vi "System_Data_Save.vi"(8 "error in":errorcluster, 11 "System Data":T1={"System"={"Active"=FALSE, "Exit"=FALSE, "Command wait"="", "Status_Time"=0, "Time_GPS"=0}, "Stepper Motor"={"Connection Reference"="", "Valid Connection"=FALSE, "Speed"=15}, "Camera Data"={"Image path"=path "", "Filenames"=[], "Filenames queue"=[]}, "Core"={"Close Panel on Exit?"=FALSE, "Current VI Reference"=refnum}} {"Stepper Motor"."Speed" scale=0.0..30.0}) -> (0 "error out":errorcluster, 3 "path":path)   [LabVIEW 2019]
uses:
  System Data.ctl
  Stepper Data.ctl
  Camera Data.ctl
  <vilib>/Utility/xml.llb/Write to XML File(string).vi
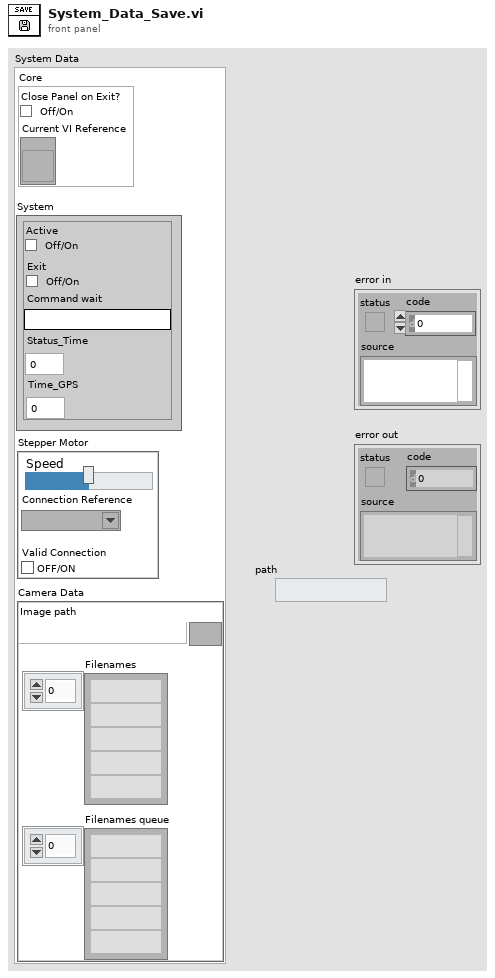
[diagram p1: front panel]
types:
  T1 = typedef "System Data.ctl" = cluster{"System":cluster{"Active":bool, "Exit":bool, "Command wait":string, "Status_Time":i32, "Time_GPS":i32}, "Stepper Motor":T2, "Camera Data":T3, "Core":cluster{"Close Panel on Exit?":bool, "Current VI Reference":refnum<vi>}}
  T2 = typedef "Stepper Data.ctl" = cluster{"Connection Reference":refnum<visa-resource-name>, "Valid Connection":bool, "Speed":i32}
  T3 = typedef "Camera Data.ctl" = cluster{"Image path":path, "Filenames":string[], "Filenames queue":string[]}
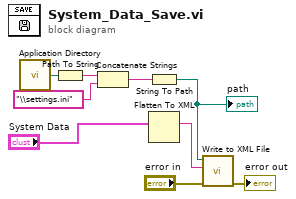
[diagram p0: block diagram]
diagram:
  n1 = call <vilib>:"Application Directory.vi"() -> ("Application Directory"=w7:path)
  n2 = Path To String(path=w7) -> (string=w8:string)
  n3 = Concatenate Strings(w8, "\\settings.ini" ("string")) -> (w5:string)
  n4 = String To Path(string=w5) -> (path=w4:path)
  "path" <- w4
  n5 = Flatten To XML(anything="System Data") -> (xml string=w9:string)
  n6 = call-poly <vilib>:"Write to XML File.vi"("error in (no error)"="error in", "XML Input"=w9, "XML File Path"=w4) -> ("error out"=→"error out":errorcluster)  [unwired: 6 in, 2 out]
